vi "setupDispCompOptimization.vi"() -> ()   [LabVIEW 2017]
uses:
  classes/Scans/Scan.lvclass
  <vilib>/gmath/NI_Gmath.lvlib
  <vilib>/Analysis/NI_AALBase.lvlib
  <vilib>/Analysis/1siggen.llb/Ramp Pattern by Samples.vi
  <vilib>/Analysis/baseanly.llb/Mean (DBL).vi
  classes/HardwareObjects/Camera/Camera.lvclass
panel:
  out "error out 3":errorcluster
  out "Image 3":T1(plugin-control)
  out "error out 2":errorcluster
  out "Image 2":T1(plugin-control)
  in  "Spectrum calibration":dbl[](array[numeric])=[1.0, 1.7154, 2.431, 3.1467, 3.8626, 4.5788, 5.2951, 6.0116, 6.7283, 7.4452, 8.1622, 8.8795, 9.5969, 10.315, 11.032, 11.75, 12.469, 13.187, 13.906, 14.624, 15.343, 16.062, 16.782, 17.501, 18.221, 18.941, 19.661, 20.381, 21.102, 21.822, 22.543, 23.264, 23.986, 24.707, 25.429, 26.15, 26.872, 27.595, 28.317, 29.04, 29.762, 30.485, 31.208, 31.932, 32.655, 33.379, 34.103, 34.827, 35.551, 36.276, 37.001, 37.725, 38.451, 39.176, 39.901, 40.627, 41.353, 42.079, 42.805, 43.531, 44.258, 44.985, 45.712, 46.439, 47.166, 47.894, 48.622, 49.35, 50.078, 50.806, 51.535, 52.263, 52.992, 53.721, 54.451, 55.18, 55.91, 56.64, 57.37, 58.1, 58.831, 59.561, 60.292, 61.023, 61.755, 62.486, 63.218, 63.95, 64.682, 65.414, 66.146, 66.879, 67.612, 68.345, 69.078, 69.811, 70.545, 71.279, 72.013, 72.747, 73.481, 74.216, 74.951, 75.686, 76.421, 77.156, 77.892, 78.628, 79.364, 80.1, 80.836, 81.573, 82.309, 83.046, 83.784, 84.521, 85.258, 85.996, 86.734, 87.472, 88.211, 88.949, 89.688, 90.427, 91.166, 91.905, 92.645, 93.385, 94.124, 94.865, 95.605, 96.345, 97.086, 97.827, 98.568, 99.31, 100.05, 100.79, 101.53, 102.28, 103.02, 103.76, 104.5, 105.25, 105.99, 106.73, 107.48, 108.22, 108.96, 109.71, 110.45, 111.2, 111.94, 112.69, 113.43, 114.18, 114.92, 115.67, 116.42, 117.16, 117.91, 118.65, 119.4, 120.15, 120.9, 121.64, 122.39, 123.14, 123.89, 124.63, 125.38, 126.13, 126.88, 127.63, 128.38, 129.13, 129.88, 130.63, 131.38, 132.13, 132.88, 133.63, 134.38, 135.13, 135.88, 136.63, 137.38, 138.14, 138.89, 139.64, 140.39, 141.15, 141.9, 142.65, 143.4, 144.16, 144.91, 145.67, 146.42, 147.17, 147.93, 148.68, 149.44, 150.19, 150.95, 151.7, 152.46, 153.22, 153.97, 154.73, 155.48, 156.24, 157.0, 157.76, 158.51, 159.27, 160.03, 160.79, 161.54, 162.3, 163.06, 163.82, 164.58, 165.34, 166.1, 166.86, 167.62, 168.38, 169.14, 169.9, 170.66, 171.42, 172.18, 172.94, 173.7, 174.47, 175.23, 175.99, 176.75, 177.51, 178.28, 179.04, 179.8, 180.57, 181.33, 182.09, 182.86, 183.62, 184.39, 185.15, 185.92, 186.68, 187.45, 188.21, 188.98, 189.74, 190.51, 191.28, 192.04, 192.81, 193.58, 194.35, 195.11, 195.88, 196.65, 197.42, 198.18, 198.95, 199.72, 200.49, 201.26, 202.03, 202.8, 203.57, 204.34, 205.11, 205.88, 206.65, 207.42, 208.19, 208.96, 209.73, 210.51, 211.28, 212.05, 212.82, 213.59, 214.37, 215.14, 215.91, 216.69, 217.46, 218.23, 219.01, 219.78, 220.56, 221.33, 222.11, 222.88, 223.66, 224.43, 225.21, 225.98, 226.76, 227.54, 228.31, 229.09, 229.87, 230.65, 231.42, 232.2, 232.98, 233.76, 234.54, 235.31, 236.09, 236.87, 237.65, 238.43, 239.21, 239.99, 240.77, 241.55, 242.33, 243.11, 243.89, 244.67, 245.46, 246.24, 247.02, 247.8, 248.58, 249.37, 250.15, 250.93, 251.71, 252.5, 253.28, 254.07, 254.85, 255.63, 256.42, 257.2, 257.99, 258.77, 259.56, 260.34, 261.13, 261.92, 262.7, 263.49, 264.27, 265.06, 265.85, 266.64, 267.42, 268.21, 269.0, 269.79, 270.58, 271.37, 272.15, 272.94, 273.73, 274.52, 275.31, 276.1, 276.89, 277.68, 278.47, 279.26, 280.06, 280.85, 281.64, 282.43, 283.22, 284.01, 284.81, 285.6, 286.39, 287.19, 287.98, 288.77, 289.57, 290.36, 291.15, 291.95, 292.74, 293.54, 294.33, 295.13, 295.92, 296.72, 297.52, 298.31, 299.11, 299.91, 300.7, 301.5, 302.3, 303.1, 303.89, 304.69, 305.49, 306.29, 307.09, 307.89, 308.69, 309.49, 310.28, 311.08, 311.88, 312.69, 313.49, 314.29, 315.09, 315.89, 316.69, 317.49, 318.29, 319.1, 319.9, 320.7, 321.5, 322.31, 323.11, 323.91, 324.72, 325.52, 326.33, 327.13, 327.94, 328.74, 329.55, 330.35, 331.16, 331.96, 332.77, 333.58, 334.38, 335.19, 336.0, 336.8, 337.61, 338.42, 339.23, 340.03, 340.84, 341.65, 342.46, 343.27, 344.08, 344.89, 345.7, 346.51, 347.32, 348.13, 348.94, 349.75, 350.56, 351.37, 352.18, 353.0, 353.81, 354.62, 355.43, 356.25, 357.06, 357.87, 358.69, 359.5, 360.31, 361.13, 361.94, 362.76, 363.57, 364.39, 365.2, 366.02, 366.83, 367.65, 368.47, 369.28, 370.1, 370.92, 371.74, 372.55, 373.37, 374.19, 375.01, 375.83, 376.64, 377.46, 378.28, 379.1, 379.92, 380.74, 381.56, 382.38, 383.2, 384.02, 384.84, 385.67, 386.49, 387.31, 388.13, 388.95, 389.78, 390.6, 391.42, 392.24, 393.07, 393.89, 394.72, 395.54, 396.36, 397.19, 398.01, 398.84, 399.66, 400.49, 401.32, 402.14, 402.97, 403.8, 404.62, 405.45, 406.28, 407.1, 407.93, 408.76, 409.59, 410.42, 411.25, 412.07, 412.9, 413.73, 414.56, 415.39, 416.22, 417.05, 417.88, 418.72, 419.55, 420.38, 421.21, 422.04, 422.87, 423.71, 424.54, 425.37, 426.21, 427.04, 427.87, 428.71, 429.54, 430.37, 431.21, 432.04, 432.88, 433.71, 434.55, 435.39, 436.22, 437.06, 437.89, 438.73, 439.57, 440.41, 441.24, 442.08, 442.92, 443.76, 444.6, 445.44, 446.27, 447.11, 447.95, 448.79, 449.63, 450.47, 451.31, 452.15, 453.0, 453.84, 454.68, 455.52, 456.36, 457.2, 458.05, 458.89, 459.73, 460.58, 461.42, 462.26, 463.11, 463.95, 464.8, 465.64, 466.49, 467.33, 468.18, 469.02, 469.87, 470.71, 471.56, 472.41, 473.25, 474.1, 474.95, 475.8, 476.65, 477.49, 478.34, 479.19, 480.04, 480.89, 481.74, 482.59, 483.44, 484.29, 485.14, 485.99, 486.84, 487.69, 488.54, 489.4, 490.25, 491.1, 491.95, 492.81, 493.66, 494.51, 495.37, 496.22, 497.07, 497.93, 498.78, 499.64, 500.49, 501.35, 502.2, 503.06, 503.92, 504.77, 505.63, 506.49, 507.34, 508.2, 509.06, 509.92, 510.77, 511.63, 512.49, 513.35, 514.21, 515.07, 515.93, 516.79, 517.65, 518.51, 519.37, 520.23, 521.09, 521.95, 522.82, 523.68, 524.54, 525.4, 526.27, 527.13, 527.99, 528.86, 529.72, 530.58, 531.45, 532.31, 533.18, 534.04, 534.91, 535.77, 536.64, 537.51, 538.37, 539.24, 540.11, 540.97, 541.84, 542.71, 543.58, 544.45, 545.31, 546.18, 547.05, 547.92, 548.79, 549.66, 550.53, 551.4, 552.27, 553.14, 554.01, 554.89, 555.76, 556.63, 557.5, 558.37, 559.25, 560.12, 560.99, 561.87, 562.74, 563.62, 564.49, 565.36, 566.24, 567.11, 567.99, 568.87, 569.74, 570.62, 571.49, 572.37, 573.25, 574.13, 575.0, 575.88, 576.76, 577.64, 578.52, 579.4, 580.27, 581.15, 582.03, 582.91, 583.79, 584.67, 585.56, 586.44, 587.32, 588.2, 589.08, 589.96, 590.85, 591.73, 592.61, 593.49, 594.38, 595.26, 596.15, 597.03, 597.91, 598.8, 599.69, 600.57, 601.46, 602.34, 603.23, 604.11, 605.0, 605.89, 606.78, 607.66, 608.55, 609.44, 610.33, 611.22, 612.11, 612.99, 613.88, 614.77, 615.66, 616.55, 617.45, 618.34, 619.23, 620.12, 621.01, 621.9, 622.79, 623.69, 624.58, 625.47, 626.37, 627.26, 628.15, 629.05, 629.94, 630.84, 631.73, 632.63, 633.52, 634.42, 635.31, 636.21, 637.11, 638.0, 638.9, 639.8, 640.7, 641.6, 642.49, 643.39, 644.29, 645.19, 646.09, 646.99, 647.89, 648.79, 649.69, 650.59, 651.49, 652.39, 653.3, 654.2, 655.1, 656.0, 656.91, 657.81, 658.71, 659.62, 660.52, 661.42, 662.33, 663.23, 664.14, 665.04, 665.95, 666.85, 667.76, 668.67, 669.57, 670.48, 671.39, 672.3, 673.2, 674.11, 675.02, 675.93, 676.84, 677.75, 678.66, 679.57, 680.48, 681.39, 682.3, 683.21, 684.12, 685.03, 685.94, 686.86, 687.77, 688.68, 689.59, 690.51, 691.42, 692.34, 693.25, 694.16, 695.08, 695.99, 696.91, 697.83, 698.74, 699.66, 700.57, 701.49, 702.41, 703.32, 704.24, 705.16, 706.08, 707.0, 707.92, 708.84, 709.75, 710.67, 711.59, 712.51, 713.44, 714.36, 715.28, 716.2, 717.12, 718.04, 718.96, 719.89, 720.81, 721.73, 722.66, 723.58, 724.5, 725.43, 726.35, 727.28, 728.2, 729.13, 730.05, 730.98, 731.91, 732.83, 733.76, 734.69, 735.62, 736.54, 737.47, 738.4, 739.33, 740.26, 741.19, 742.12, 743.05, 743.98, 744.91, 745.84, 746.77, 747.7, 748.63, 749.56, 750.5, 751.43, 752.36, 753.3, 754.23, 755.16, 756.1, 757.03, 757.97, 758.9, 759.84, 760.77, 761.71, 762.64, 763.58, 764.52, 765.45, 766.39, 767.33, 768.27, 769.21, 770.14, 771.08, 772.02, 772.96, 773.9, 774.84, 775.78, 776.72, 777.66, 778.61, 779.55, 780.49, 781.43, 782.37, 783.32, 784.26, 785.2, 786.15, 787.09, 788.04, 788.98, 789.93, 790.87, 791.82, 792.76, 793.71, 794.65, 795.6, 796.55, 797.5, 798.44, 799.39, 800.34, 801.29, 802.24, 803.19, 804.14, 805.09, 806.04, 806.99, 807.94, 808.89, 809.84, 810.79, 811.74, 812.7, 813.65, 814.6, 815.56, 816.51, 817.46, 818.42, 819.37, 820.33, 821.28, 822.24, 823.19, 824.15, 825.1, 826.06, 827.02, 827.98, 828.93, 829.89, 830.85, 831.81, 832.77, 833.73, 834.69, 835.65, 836.61, 837.57, 838.53, 839.49, 840.45, 841.41, 842.37, 843.34, 844.3, 845.26, 846.22, 847.19, 848.15, 849.12, 850.08, 851.05, 852.01, 852.98, 853.94, 854.91, 855.87, 856.84, 857.81, 858.78, 859.74, 860.71, 861.68, 862.65, 863.62, 864.59, 865.56, 866.53, 867.5, 868.47, 869.44, 870.41, 871.38, 872.35, 873.32, 874.3, 875.27, 876.24, 877.22, 878.19, 879.16, 880.14, 881.11, 882.09, 883.06, 884.04, 885.02, 885.99, 886.97, 887.95, 888.92, 889.9, 890.88, 891.86, 892.84, 893.81, 894.79, 895.77, 896.75, 897.73, 898.71, 899.69, 900.68, 901.66, 902.64, 903.62, 904.6, 905.59, 906.57, 907.55, 908.54, 909.52, 910.51, 911.49, 912.48, 913.46, 914.45, 915.43, 916.42, 917.41, 918.39, 919.38, 920.37, 921.36, 922.35, 923.33, 924.32, 925.31, 926.3, 927.29, 928.28, 929.27, 930.27, 931.26, 932.25, 933.24, 934.23, 935.23, 936.22, 937.21, 938.21, 939.2, 940.19, 941.19, 942.18, 943.18, 944.18, 945.17, 946.17, 947.16, 948.16, 949.16, 950.16, 951.16, 952.15, 953.15, 954.15, 955.15, 956.15, 957.15, 958.15, 959.15, 960.15, 961.16, 962.16, 963.16, 964.16, 965.16, 966.17, 967.17, 968.18, 969.18, 970.18, 971.19, 972.19, 973.2, 974.21, 975.21, 976.22, 977.23, 978.23, 979.24, 980.25, 981.26, 982.27, 983.27, 984.28, 985.29, 986.3, 987.31, 988.32, 989.34, 990.35, 991.36, 992.37, 993.38, 994.4, 995.41, 996.42, 997.44, 998.45, 999.46, 1000.5, 1001.5, 1002.5, 1003.5, 1004.5, 1005.6, 1006.6, 1007.6, 1008.6, 1009.6, 1010.6, 1011.7, 1012.7, 1013.7, 1014.7, 1015.7, 1016.8, 1017.8, 1018.8, 1019.8, 1020.8, 1021.9, 1022.9, 1023.9, 1024.9, 1026.0, 1027.0, 1028.0, 1029.0, 1030.1, 1031.1, 1032.1, 1033.1, 1034.2, 1035.2, 1036.2, 1037.2, 1038.3, 1039.3, 1040.3, 1041.4, 1042.4, 1043.4, 1044.4, 1045.5, 1046.5, 1047.5, 1048.6, 1049.6, 1050.6, 1051.7, 1052.7, 1053.7, 1054.8, 1055.8, 1056.8, 1057.9, 1058.9, 1059.9, 1061.0, 1062.0, 1063.0, 1064.1, 1065.1, 1066.2, 1067.2, 1068.2, 1069.3, 1070.3, 1071.4, 1072.4, 1073.4, 1074.5, 1075.5, 1076.6, 1077.6, 1078.6, 1079.7, 1080.7, 1081.8, 1082.8, 1083.9, 1084.9, 1085.9, 1087.0, 1088.0, 1089.1, 1090.1, 1091.2, 1092.2, 1093.3, 1094.3, 1095.4, 1096.4, 1097.5, 1098.5, 1099.6, 1100.6, 1101.7, 1102.7, 1103.8, 1104.8, 1105.9, 1106.9, 1108.0, 1109.0, 1110.1, 1111.1, 1112.2, 1113.2, 1114.3, 1115.3, 1116.4, 1117.4, 1118.5, 1119.6, 1120.6, 1121.7, 1122.7, 1123.8, 1124.8, 1125.9, 1127.0, 1128.0, 1129.1, 1130.1, 1131.2, 1132.3, 1133.3, 1134.4, 1135.4, 1136.5, 1137.6, 1138.6, 1139.7, 1140.8, 1141.8, 1142.9, 1144.0, 1145.0, 1146.1, 1147.1, 1148.2, 1149.3, 1150.3, 1151.4, 1152.5, 1153.6, 1154.6, 1155.7, 1156.8, 1157.8, 1158.9, 1160.0, 1161.0, 1162.1, 1163.2, 1164.3, 1165.3, 1166.4, 1167.5, 1168.5, 1169.6, 1170.7, 1171.8, 1172.8, 1173.9, 1175.0, 1176.1, 1177.2, 1178.2, 1179.3, 1180.4, 1181.5, 1182.5, 1183.6, 1184.7, 1185.8, 1186.9, 1187.9, 1189.0, 1190.1, 1191.2, 1192.3, 1193.3, 1194.4, 1195.5, 1196.6, 1197.7, 1198.8, 1199.9, 1200.9, 1202.0, 1203.1, 1204.2, 1205.3, 1206.4, 1207.5, 1208.5, 1209.6, 1210.7, 1211.8, 1212.9, 1214.0, 1215.1, 1216.2, 1217.3, 1218.4, 1219.4, 1220.5, 1221.6, 1222.7, 1223.8, 1224.9, 1226.0, 1227.1, 1228.2, 1229.3, 1230.4, 1231.5, 1232.6, 1233.7, 1234.8, 1235.9, 1237.0, 1238.1, 1239.2, 1240.3, 1241.4, 1242.5, 1243.6, 1244.7, 1245.8, 1246.9, 1248.0, 1249.1, 1250.2, 1251.3, 1252.4, 1253.5, 1254.6, 1255.7, 1256.8, 1257.9, 1259.0, 1260.1, 1261.2, 1262.3, 1263.5, 1264.6, 1265.7, 1266.8, 1267.9, 1269.0, 1270.1, 1271.2, 1272.3, 1273.4, 1274.6, 1275.7, 1276.8, 1277.9, 1279.0, 1280.1, 1281.2, 1282.4, 1283.5, 1284.6, 1285.7, 1286.8, 1287.9, 1289.1, 1290.2, 1291.3, 1292.4, 1293.5, 1294.6, 1295.8, 1296.9, 1298.0, 1299.1, 1300.2, 1301.4, 1302.5, 1303.6, 1304.7, 1305.9, 1307.0, 1308.1, 1309.2, 1310.4, 1311.5, 1312.6, 1313.7, 1314.9, 1316.0, 1317.1, 1318.3, 1319.4, 1320.5, 1321.6, 1322.8, 1323.9, 1325.0, 1326.2, 1327.3, 1328.4, 1329.6, 1330.7, 1331.8, 1333.0, 1334.1, 1335.2, 1336.4, 1337.5, 1338.6, 1339.8, 1340.9, 1342.0, 1343.2, 1344.3, 1345.5, 1346.6, 1347.7, 1348.9, 1350.0, 1351.2, 1352.3, 1353.4, 1354.6, 1355.7, 1356.9, 1358.0, 1359.2, 1360.3, 1361.4, 1362.6, 1363.7, 1364.9, 1366.0, 1367.2, 1368.3, 1369.5, 1370.6, 1371.8, 1372.9, 1374.1, 1375.2, 1376.4, 1377.5, 1378.7, 1379.8, 1381.0, 1382.1, 1383.3, 1384.4, 1385.6, 1386.7, 1387.9, 1389.0, 1390.2, 1391.4, 1392.5, 1393.7, 1394.8, 1396.0, 1397.1, 1398.3, 1399.5, 1400.6, 1401.8, 1402.9, 1404.1, 1405.3, 1406.4, 1407.6, 1408.7, 1409.9, 1411.1, 1412.2, 1413.4, 1414.6, 1415.7, 1416.9, 1418.1, 1419.2, 1420.4, 1421.6, 1422.7, 1423.9, 1425.1, 1426.2, 1427.4, 1428.6, 1429.7, 1430.9, 1432.1, 1433.3, 1434.4, 1435.6, 1436.8, 1438.0, 1439.1, 1440.3, 1441.5, 1442.7, 1443.8, 1445.0, 1446.2, 1447.4, 1448.5, 1449.7, 1450.9, 1452.1, 1453.3, 1454.4, 1455.6, 1456.8, 1458.0, 1459.2, 1460.3, 1461.5, 1462.7, 1463.9, 1465.1, 1466.3, 1467.4, 1468.6, 1469.8, 1471.0, 1472.2, 1473.4, 1474.6, 1475.8, 1476.9, 1478.1, 1479.3, 1480.5, 1481.7, 1482.9, 1484.1, 1485.3, 1486.5, 1487.7, 1488.9, 1490.1, 1491.3, 1492.4, 1493.6, 1494.8, 1496.0, 1497.2, 1498.4, 1499.6, 1500.8, 1502.0, 1503.2, 1504.4, 1505.6, 1506.8, 1508.0, 1509.2, 1510.4, 1511.6, 1512.8, 1514.0, 1515.2, 1516.4, 1517.7, 1518.9, 1520.1, 1521.3, 1522.5, 1523.7, 1524.9, 1526.1, 1527.3, 1528.5, 1529.7, 1530.9, 1532.1, 1533.4, 1534.6, 1535.8, 1537.0, 1538.2, 1539.4, 1540.6, 1541.9, 1543.1, 1544.3, 1545.5, 1546.7, 1547.9, 1549.1, 1550.4, 1551.6, 1552.8, 1554.0, 1555.2, 1556.5, 1557.7, 1558.9, 1560.1, 1561.4, 1562.6, 1563.8, 1565.0, 1566.2, 1567.5, 1568.7, 1569.9, 1571.1, 1572.4, 1573.6, 1574.8, 1576.1, 1577.3, 1578.5, 1579.7, 1581.0, 1582.2, 1583.4, 1584.7, 1585.9, 1587.1, 1588.4, 1589.6, 1590.8, 1592.1, 1593.3, 1594.5, 1595.8, 1597.0, 1598.3, 1599.5, 1600.7, 1602.0, 1603.2, 1604.4, 1605.7, 1606.9, 1608.2, 1609.4, 1610.7, 1611.9, 1613.1, 1614.4, 1615.6, 1616.9, 1618.1, 1619.4, 1620.6, 1621.9, 1623.1, 1624.4, 1625.6, 1626.8, 1628.1, 1629.3, 1630.6, 1631.8, 1633.1, 1634.4, 1635.6, 1636.9, 1638.1, 1639.4, 1640.6, 1641.9, 1643.1, 1644.4, 1645.6, 1646.9, 1648.2, 1649.4, 1650.7, 1651.9, 1653.2, 1654.5, 1655.7, 1657.0, 1658.2, 1659.5, 1660.8, 1662.0, 1663.3, 1664.6, 1665.8, 1667.1, 1668.4, 1669.6, 1670.9, 1672.2, 1673.4, 1674.7, 1676.0, 1677.2, 1678.5, 1679.8, 1681.0, 1682.3, 1683.6, 1684.9, 1686.1, 1687.4, 1688.7, 1690.0, 1691.2, 1692.5, 1693.8, 1695.1, 1696.3, 1697.6, 1698.9, 1700.2, 1701.5, 1702.7, 1704.0, 1705.3, 1706.6, 1707.9, 1709.1, 1710.4, 1711.7, 1713.0, 1714.3, 1715.6, 1716.8, 1718.1, 1719.4, 1720.7, 1722.0, 1723.3, 1724.6, 1725.9, 1727.2, 1728.5, 1729.7, 1731.0, 1732.3, 1733.6, 1734.9, 1736.2, 1737.5, 1738.8, 1740.1, 1741.4, 1742.7, 1744.0, 1745.3, 1746.6, 1747.9, 1749.2, 1750.5, 1751.8, 1753.1, 1754.4, 1755.7, 1757.0, 1758.3, 1759.6, 1760.9, 1762.2, 1763.5, 1764.8, 1766.1, 1767.4, 1768.7, 1770.1, 1771.4, 1772.7, 1774.0, 1775.3, 1776.6, 1777.9, 1779.2, 1780.5, 1781.9, 1783.2, 1784.5, 1785.8, 1787.1, 1788.4, 1789.8, 1791.1, 1792.4, 1793.7, 1795.0, 1796.3, 1797.7, 1799.0, 1800.3, 1801.6, 1803.0, 1804.3, 1805.6, 1806.9, 1808.3, 1809.6, 1810.9, 1812.2, 1813.6, 1814.9, 1816.2, 1817.5, 1818.9, 1820.2, 1821.5, 1822.9, 1824.2, 1825.5, 1826.9, 1828.2, 1829.5, 1830.9, 1832.2, 1833.5, 1834.9, 1836.2, 1837.6, 1838.9, 1840.2, 1841.6, 1842.9, 1844.2, 1845.6, 1846.9, 1848.3, 1849.6, 1851.0, 1852.3, 1853.7, 1855.0, 1856.3, 1857.7, 1859.0, 1860.4, 1861.7, 1863.1, 1864.4, 1865.8, 1867.1, 1868.5, 1869.8, 1871.2, 1872.5, 1873.9, 1875.2, 1876.6, 1878.0, 1879.3, 1880.7, 1882.0, 1883.4, 1884.7, 1886.1, 1887.5, 1888.8, 1890.2, 1891.5, 1892.9, 1894.3, 1895.6, 1897.0, 1898.4, 1899.7, 1901.1, 1902.5, 1903.8, 1905.2, 1906.6, 1907.9, 1909.3, 1910.7, 1912.0, 1913.4, 1914.8, 1916.2, 1917.5, 1918.9, 1920.3, 1921.7, 1923.0, 1924.4, 1925.8, 1927.2, 1928.5, 1929.9, 1931.3, 1932.7, 1934.1, 1935.4, 1936.8, 1938.2, 1939.6, 1941.0, 1942.4, 1943.7, 1945.1, 1946.5, 1947.9, 1949.3, 1950.7, 1952.1, 1953.5, 1954.8, 1956.2, 1957.6, 1959.0, 1960.4, 1961.8, 1963.2, 1964.6, 1966.0, 1967.4, 1968.8, 1970.2, 1971.6, 1973.0, 1974.4, 1975.8, 1977.2, 1978.6, 1980.0, 1981.4, 1982.8, 1984.2, 1985.6, 1987.0, 1988.4, 1989.8, 1991.2, 1992.6, 1994.0, 1995.4, 1996.8, 1998.2, 1999.7, 2001.1, 2002.5, 2003.9, 2005.3, 2006.7, 2008.1, 2009.5, 2011.0, 2012.4, 2013.8, 2015.2, 2016.6, 2018.1, 2019.5, 2020.9, 2022.3, 2023.7, 2025.2, 2026.6, 2028.0, 2029.4, 2030.9, 2032.3, 2033.7, 2035.1, 2036.6, 2038.0, 2039.4, 2040.8, 2042.3, 2043.7, 2045.1, 2046.6]
  in  "Camera in":refnum<class "Camera.lvclass">
  out "P":dbl[](array[numeric])
  out "bg":dbl[](array[numeric])
  out "Image":T1(plugin-control)
  out "error out":errorcluster
  out "Y offset (degrees)":dbl
  out "Y FOV (degrees)":dbl
  out "X offset (degrees)":dbl
  out "X FOV (degrees)":dbl
  out "Total B-Scans":dbl
  out "Total A-scans per volume":dbl
  out "Total A-scans per frame":dbl
  out "Scan Pattern":string
  out "Scan Angle (degrees)":dbl
  out "Repeat B scans":dbl
  out "C scans":dbl
  out "Bidirectional":bool
  out "B scans":dbl
  out "Angio Mode":string
  out "A scans":dbl
  in  "debug":bool=TRUE
  out "Scan out":refnum<class "Scan.lvclass">
  in  "Scan type":refnum<class "Scan.lvclass">
  out "Most recent scan fname":string
  in  "File Ctrl":T2={"Subject ID"="noise", "Eye"=FALSE, "Output Path"=path "F:/img/2019.11.13-DM_180402/OCTA/2019_11_13_OS/Raw", "String"="OS", "String 2"="OD"}
  out "Dispersion Ctrl 2":cluster{"C2":dbl, "C3":dbl}
  in  "Dispersion Ctrl":cluster{"C2":dbl, "C3":dbl}
  # "exp(i*C2*(k-k0)^2 + C3*(k-k0)^3)"
  # "exp(i*C2*(k-k0)^2 + C3*(k-k0)^3)"
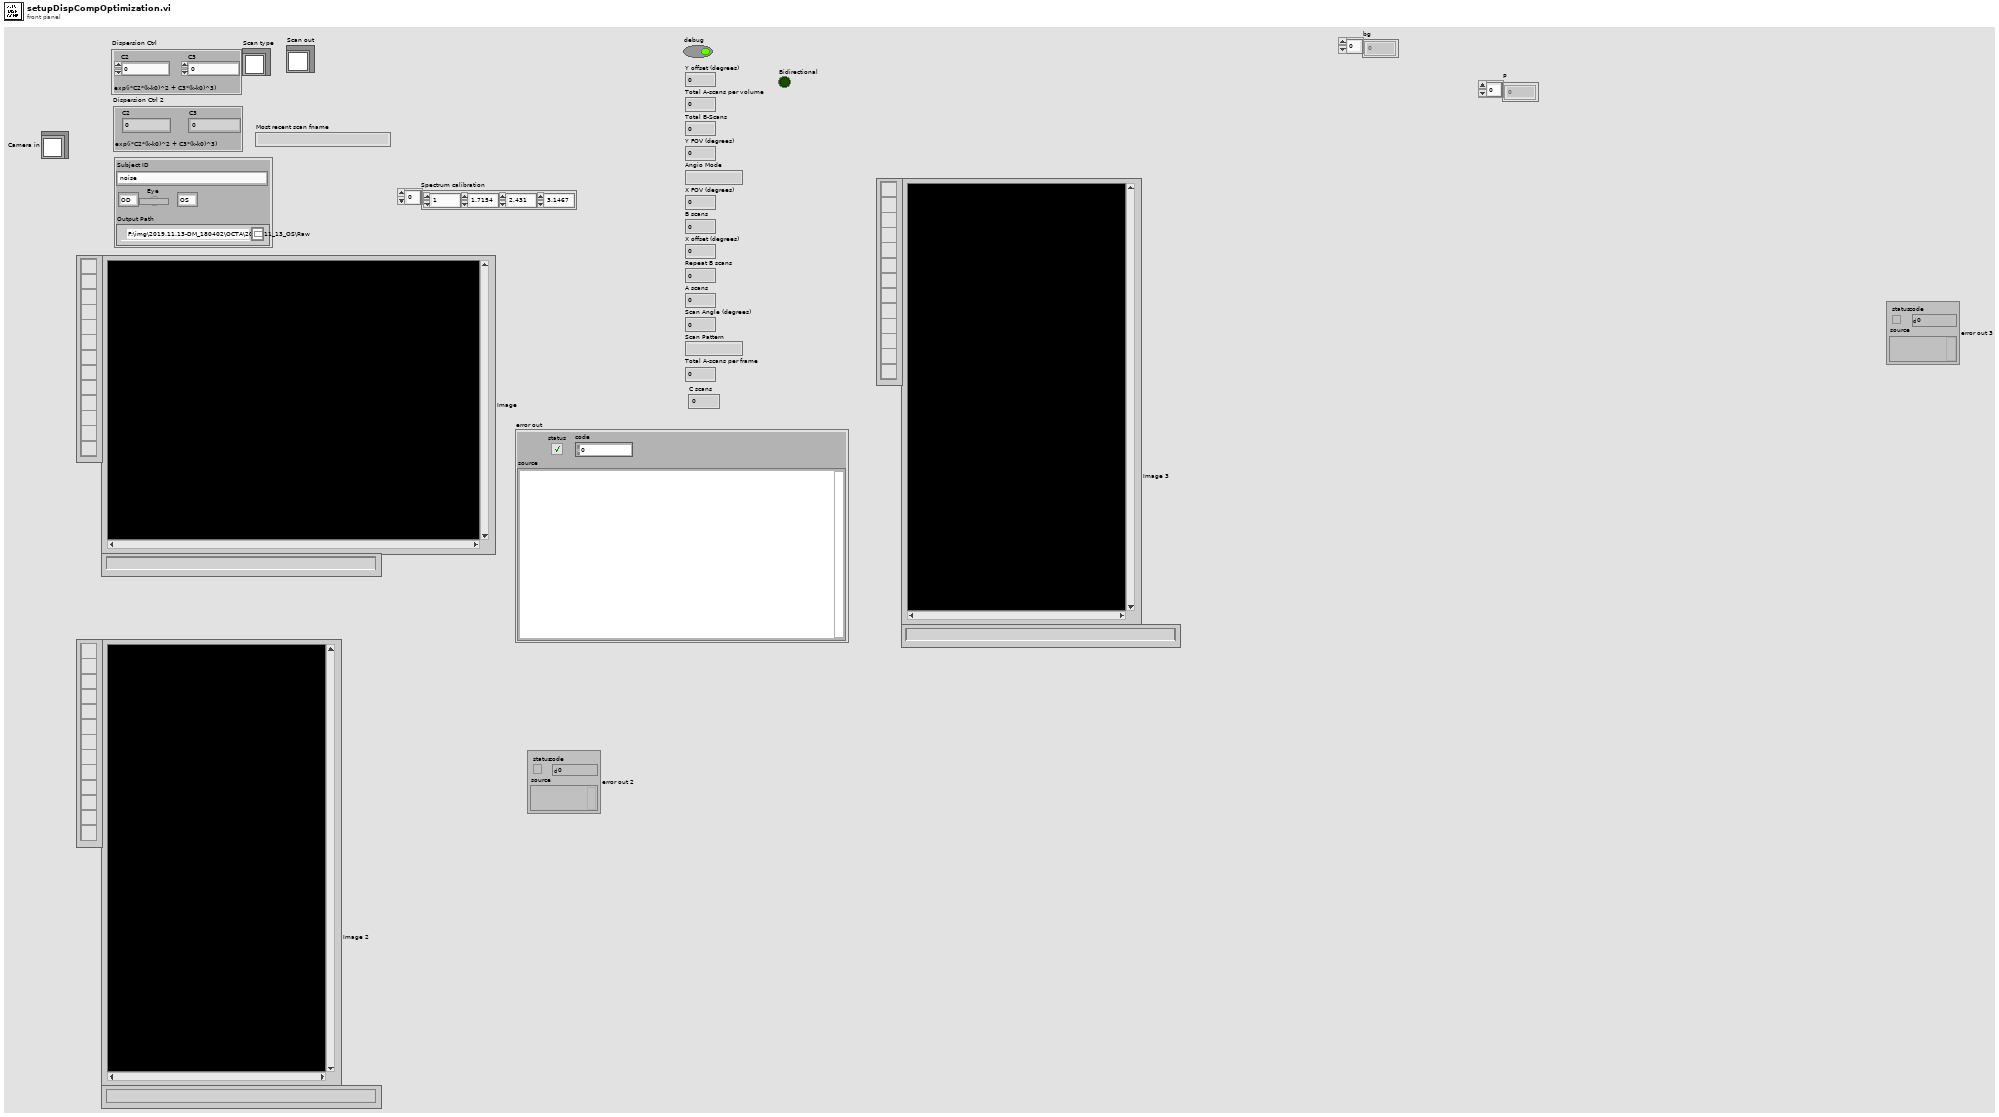
[diagram p1: front panel]
types:
  T1 = typedef "IMAQ Image.ctl" = refnum<image>
  T2 = cluster{"Subject ID":string, "Eye":bool, "Output Path":path, "String":string, "String 2":string}
  T3 = typedef "Image Type" = u32
  T4 = enum16{"big-endian, network order", "native, host order", "little-endian"}
  T5 = enum16{"open", "replace", "create", "open or create", "replace or create", "replace or create with confirmation"}
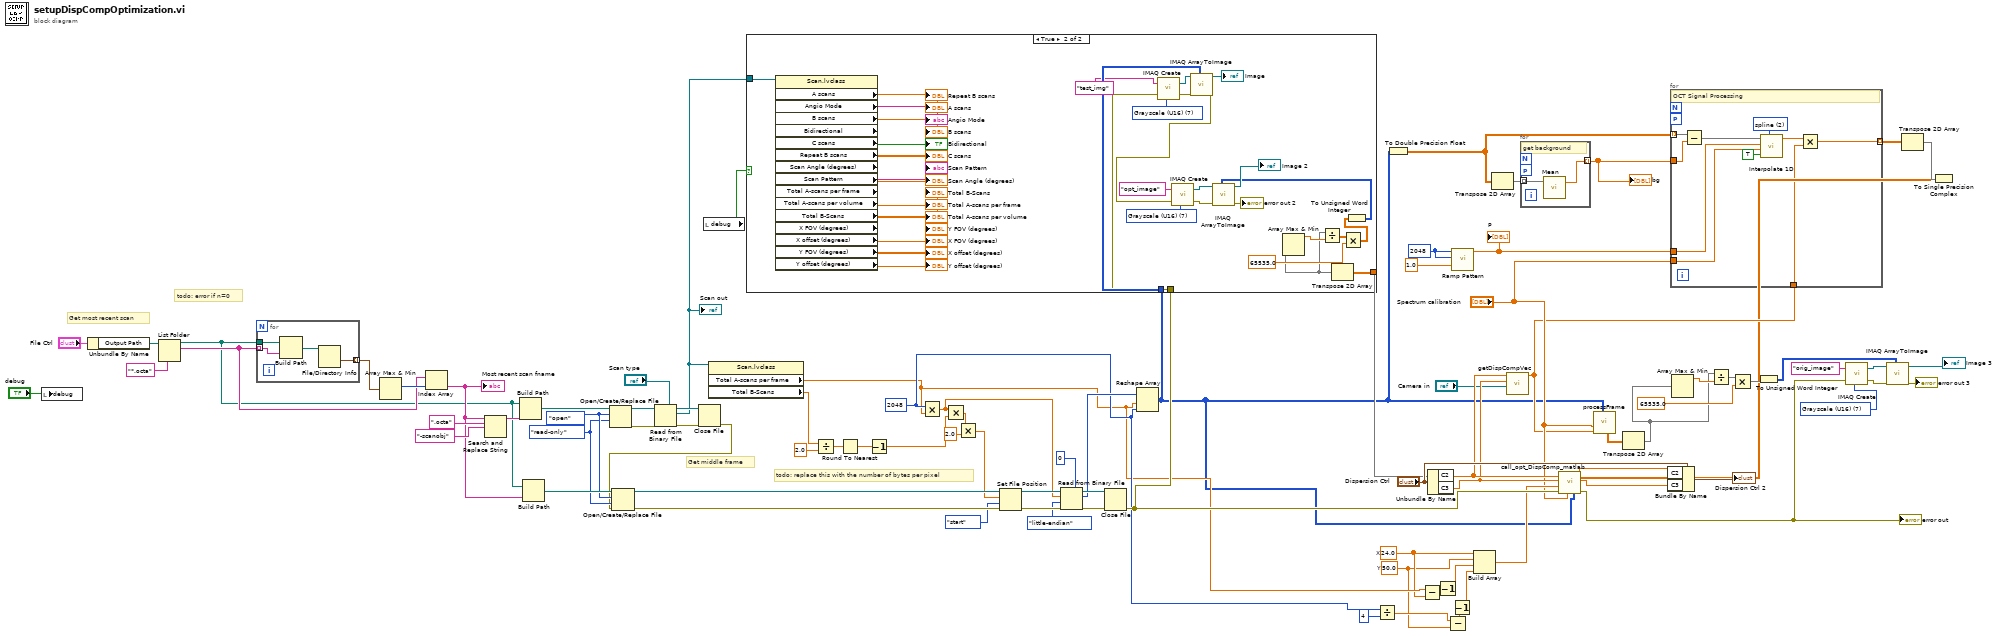
[diagram p0: block diagram]
diagram:
  w3 = T3 7 items=["Grayscale (U8)", "Grayscale (I16)", "Grayscale (SGL)", "Complex (CSG)", "RGB (U32)", "HSL (U32)", "RGB (U64)", "Grayscale (U16)"] ("Image Type")
  w33 = 2048 ("samples")
  w34 = 50.0  # Y
  w36 = 24.0  # X
  w41 = 2048 ("dimension size")
  w68 = enum16{"read/write", "read-only", "write-only"}."read-only" ("access (0:read/write)")
  w69 = T5."open" ("operation (0:open)")
  # "Get middle frame"
  # "todo: replace this with the number of bytes per pixel"
  # "todo: error if n=0"
  # "Get most recent scan"
  n1 = local write "debug"("debug") -> ()
  n2 = Unbundle By Name("File Ctrl") -> ("Output Path"=w88:path)
  n3 = List Folder(path=w88, pattern="*.octa") -> (path out=w71:path, filenames=w84:string[])  [unwired: 2 in, 2 out]
  n4 = for {
    tunnel: w84 -> [w92] mode=indexing
    tunnel: w71 -> [w93]
    tunnel: [w90] -> w86 mode=indexing
    n5 = Build Path(base path=w93, name or relative path=w92) -> (appended path=w91:path)
    n6 = File/Directory Info(path=w91) -> (last mod=w90:timestamp)  [unwired: 1 in, 6 out]
  }
  n7 = Array Max & Min(array=w86) -> (max index (indices)=w85:i32)  [unwired: 3 out]
  n8 = Index Array(array=w84, index=w85) -> (element=w72:string)
  "Most recent scan fname" <- w72
  n9 = Search and Replace String(input string=w72, search string=".octa", replace string="-scanobj" ("replace string (\"\")")) -> (result string=w81:string)  [unwired: 5 in, 3 out]
  n10 = Build Path(base path=w71, name or relative path=w81) -> (appended path=w80:path)
  n11 = Build Path(base path=w71, name or relative path=w72) -> (appended path=w70:path)
  n12 = Open/Create/Replace File(file path (use dialog)=w80, operation (0:open)=w69, access (0:read/write)=w68) -> (refnum out=w79:refnum<file>, error out=w74:errorcluster)  [unwired: 3 in, 1 out]
  n13 = Read from Binary File(5:"Scan type", 8:w74, 11:w79) -> (0:w73:errorcluster, 2:w67:refnum<class "Scan.lvclass">, 3:w75:refnum<file>)  [unwired: 3 in, 1 out]
  "Scan out" <- w67
  n14 = Close File(refnum=w75, error in=w73) -> (error out=w47:errorcluster)  [unwired: 1 out]
  n15 = Open/Create/Replace File(file path (use dialog)=w70, error in=w47, operation (0:open)=w69, access (0:read/write)=w68) -> (refnum out=w62:refnum<file>, error out=w59:errorcluster)  [unwired: 2 in, 1 out]
  n16 = local read "debug"() -> (w76:bool)
  n17 = property class="Scan.lvclass"(reference=w67) -> ("Total A-scans per frame"=w37:dbl, "Total B-Scans"=w66:dbl)  [unwired: 1 in, 2 out]
  n18 = Divide(x=w66, y=2.0) -> (x/y=w64:dbl)
  n19 = Round To Nearest(number=w64) -> (nearest integer value=w63:dbl)
  n20 = Decrement(x=w63) -> (x-1=w48:dbl)
  n21 = Multiply(x=w41, y=w37) -> (x*y=w50:dbl)
  n22 = Multiply(x=w50, y=w48) -> (x*y=w51:dbl)
  n23 = Multiply(x=w51, y=2.0) -> (x*y=w55:dbl)
  n24 = Set File Position(offset (in bytes) (0)=w55, refnum=w62, from (0:start)=enum16{"start", "end", "current"}."start", error in=w59) -> (refnum out=w61:refnum<file>, error out=w58:errorcluster)
  n25 = Read from Binary File(5:u16 0, 8:w58, 9:T4."little-endian" ("byte order (0:big-endian, network order)"), 10:w50, 11:w61) -> (0:w57:errorcluster, 2:w49:u16[], 3:w60:refnum<file>)  [unwired: 1 in, 1 out]
  n26 = Close File(refnum=w60, error in=w57) -> (error out=w46:errorcluster)  [unwired: 1 out]
  n27 = Reshape Array(w49, w37, w41) -> (w17:u16[][])
  n28 = Divide(x=w41, y=4) -> (x/y=w39:dbl)
  n29 = To Double Precision Float(number=w17) -> (double precision float=w26:dbl[][])
  n30 = Subtract(x=w37, y=w36) -> (x-y=w38:dbl)
  n31 = Unbundle By Name("Dispersion Ctrl") -> ("C2"=w29:dbl, "C3"=w28:dbl)
  n32 = Decrement(x=w38) -> (x-1=w25:dbl)
  n33 = Subtract(x=w39, y=w34) -> (x-y=w35:dbl)
  n34 = Decrement(x=w35) -> (x-1=w24:dbl)
  n35 = call-poly <vilib>:"Ramp Pattern.vi"("start"=1.0, "end"=w33, "samples"=w33) -> ("Ramp Pattern"=w31:dbl[])  [unwired: 7 in, 1 out]
  "P" <- w31
  n36 = Build Array(w36, w34, w25, w24) -> (w21:dbl[])
  n37 = Transpose 2D Array(2D array=w26) -> (transposed array=w30:dbl[][])
  n38 = call "getDispCompVec.vi"("Camera in"="Camera in", "C3"=w28, "C2"=w29) -> ("Gc"=w18:cdb[])  [unwired: 8 in]
  n39 = for {
    tunnel: w30 -> [w94] mode=indexing
    tunnel: [w95] -> w23 mode=indexing
    workers-P: _ -> [_]
    # "get background"
    n40 = call-poly <vilib>:"Mean.vi"("X"=w94) -> ("mean"=w95:dbl)  [unwired: 1 out]
  }
  "bg" <- w23
  n41 = call "processFrame.vi"("Image"=w17, "Gc"=w18, "wavenumber vector"="Spectrum calibration") -> ("Image out"=w13:dbl[][])  [unwired: 8 in]
  n42 = Transpose 2D Array(2D array=w13) -> (transposed array=w12:dbl[][])
  n43 = for {
    tunnel: w26 -> [w105] mode=indexing
    tunnel: w23 -> [w104]
    tunnel: w31 -> [w102]
    tunnel: "Spectrum calibration" -> [w101]
    workers-P: _ -> [_]
    tunnel: w18 -> [w97]
    tunnel: [w96] -> w22 mode=indexing
    w99 = 2 items=["nearest", "linear", "spline", "cubic Hermite", "Lagrange"] ("method")
    # "OCT Signal Processing"
    n44 = Subtract(x=w105, y=w104) -> (x-y=w103:dbl[])
    n45 = call <vilib>:"Interpolate 1D.vi"("method"=w99, "X is monotonic"=TRUE, "xi"=w101, "X"=w102, "Y"=w103) -> ("yi"=w98:dbl[])  [unwired: 4 in, 2 out]
    n46 = Multiply(x=w98, y=w97) -> (x*y=w96:cdb[])
  }
  n47 = Array Max & Min(array=w12) -> (max value=w16:dbl)  [unwired: 3 out]
  n48 = Divide(x=w12, y=w16) -> (x/y=w15:dbl[][])
  n49 = Multiply(x=w15, y=65535.0) -> (x*y=w11:dbl[][])
  n50 = To Unsigned Word Integer(number=w11) -> (unsigned 16bit integer=w5:u16[][])
  n51 = Transpose 2D Array(2D array=w22) -> (transposed array=w2:cdb[][])
  n52 = To Single Precision Complex(1:w2) -> (0:w1:csg[][])
  n53 = call "call_opt_DispComp_matlab.vi"(4:w17, 6:"Spectrum calibration", 7:w1, "error in"=w46, 9:w21, 10:w28, "Raw image"=w29) -> ("error out"=w6:errorcluster, "C2 out"=w43:dbl, "dispCompPhasor"=w44:cdb[], 5:w20)  [unwired: 1 out]
  "error out" <- w6
  n54 = case shown="True" w76 {
    tunnel: w67 -> [_ w142]
    tunnel: w17 -> [_ w126]
    tunnel: w46 -> [_ w124]
    tunnel: w20 -> [_ w112]
    frame False {
    }
    frame True {
      w118 = T3 7 items=["Grayscale (U8)", "Grayscale (I16)", "Grayscale (SGL)", "Complex (CSG)", "RGB (U32)", "HSL (U32)", "RGB (U64)", "Grayscale (U16)"] ("Image Type")
      w120 = T3 7 items=["Grayscale (U8)", "Grayscale (I16)", "Grayscale (SGL)", "Complex (CSG)", "RGB (U32)", "HSL (U32)", "RGB (U64)", "Grayscale (U16)"] ("Image Type")
      n55 = property class="Scan.lvclass"(reference=w142) -> ("A scans"=→"A scans":dbl, "Angio Mode"=→"Angio Mode":string, "B scans"=→"B scans":dbl, "Bidirectional"=→"Bidirectional":bool, "C scans"=→"C scans":dbl, "Repeat B scans"=→"Repeat B scans":dbl, "Scan Angle (degrees)"=→"Scan Angle (degrees)":dbl, "Scan Pattern"=→"Scan Pattern":string, "Total A-scans per frame"=→"Total A-scans per frame":dbl, "Total A-scans per volume"=→"Total A-scans per volume":dbl, "Total B-Scans"=→"Total B-Scans":dbl, "X FOV (degrees)"=→"X FOV (degrees)":dbl, "X offset (degrees)"=→"X offset (degrees)":dbl, "Y FOV (degrees)"=→"Y FOV (degrees)":dbl, "Y offset (degrees)"=→"Y offset (degrees)":dbl)  [unwired: 1 in, 2 out]
      n56 = call "IMAQ Create"("Image Name"="test_img", "Image Type"=w120, "error in (no error)"=w124) -> ("New Image"=w123:T1, "error out"=w122:errorcluster)  [unwired: 2 in]
      n57 = call "IMAQ ArrayToImage"("Image Pixels (U16)"=w126, "error in (no error)"=w122, "Image"=w123) -> ("error out"=w115:errorcluster, "Image Out"=→"Image":T1)  [unwired: 7 in]
      n58 = call "IMAQ Create"("Image Name"="opt_image", "Image Type"=w118, "error in (no error)"=w115) -> ("New Image"=w117:T1, "error out"=w114:errorcluster)  [unwired: 2 in]
      n59 = Transpose 2D Array(2D array=w112) -> (transposed array=w106:dbl[][])
      n60 = Array Max & Min(array=w106) -> (max value=w111:dbl)  [unwired: 3 out]
      n61 = Divide(x=w106, y=w111) -> (x/y=w110:dbl[][])
      n62 = Multiply(x=w110, y=65535.0) -> (x*y=w108:dbl[][])
      n63 = To Unsigned Word Integer(number=w108) -> (unsigned 16bit integer=w107:u16[][])
      n64 = call "IMAQ ArrayToImage"("Image Pixels (U16)"=w107, "error in (no error)"=w114, "Image"=w117) -> ("error out"=→"error out 2":errorcluster, "Image Out"=→"Image 2":T1)  [unwired: 7 in]
    }
  }
  n65 = Bundle By Name(cluster="Dispersion Ctrl", "C2"=w44, "C3"=w43) -> (→"Dispersion Ctrl 2":cluster{"C2":dbl, "C3":dbl})
  n66 = call "IMAQ Create"("Image Name"="orig_image", "Image Type"=w3, "error in (no error)"=w6) -> ("New Image"=w9:T1, "error out"=w8:errorcluster)  [unwired: 2 in]
  n67 = call "IMAQ ArrayToImage"("Image Pixels (U16)"=w5, "error in (no error)"=w8, "Image"=w9) -> ("error out"=→"error out 3":errorcluster, "Image Out"=→"Image 3":T1)  [unwired: 7 in]
